vi "BuildCustomDashBoardData.vi"   [LabVIEW 2013]
doc: "This VI builds data and sends it back to the dashboard PC program. By default it sends back the raw values for the first analog, digital, and solenoid module. Modify it to send back the data you want to view. Consider adding higher level data to the Dashboard Datatype.ctl and to this VI. Then update the Dashboard to display the data however you like.\n\nThis software is licensed. Open the labview\\readme\\WPI Robotics Library Open Source License.txt file for more information."
uses:
  <vilib>/Rock Robotics/WPI/DriverStation/WPI_DriverStationDigitalData.ctl
  typedefs/subStates.ctl
  I2C Accelerometer/ADXL345 I2C Axis.ctl
  typedefs/fg_typedef.ctl
  <vilib>/NI_Real-Time Target Support.lvlib
  typedefs/Dashboard Datatype.ctl
  typedefs/DashboardEnable.ctl
  typedefs/custom dash data.ctl
types:
  T1 = typedef "custom dash data.ctl" = cluster{"doubles":cluster{"Front Shooter Speed":dbl, "Arm Rate":dbl, "Arm Distance":dbl, "Right Distance":dbl, "Right Rate":dbl, "Left Rate":dbl, "Left Distance":dbl, "Auger Distance":dbl, "Auger Rate":dbl, "Shooter Bias":dbl, "Rear Shooter Speed":dbl}, "substates":cluster{"Shooter Belt":T2, "Shooter Arm":T2, "Shooter":T2, "Auger ":T2, "Drive":T2}, "bools":cluster{"Auger Safety":bool, "Arm Safety":bool, "Arm Limit":bool}, "Performance":cluster{"CPU Usage":dbl, "Vision mSPI":u32, "Main mSPI":u32}, "Target Info":cluster{"Left":i32, "Top":i32, "Right":i32, "Bottom":i32, "Target CoM X":dbl, "Target CoM Y":dbl}}
  T2 = typedef "subStates.ctl" = enum16{"null", "wait", "driver control", "auto", "manual override", "hold position", "rotate", "pickup", "pass", "load", "goto shoot", "shoot", "end"}
  T3 = typedef "DashboardEnable.ctl" = cluster{"Analog Module 1":bool[], "Analog Module 2":bool[], "Digital Module 1":bool, "Digital Module 2":bool, "Solenoid Module":bool}
  T4 = typedef "Dashboard Datatype.ctl" = cluster{cluster{"AnalogModule[0]":cluster{"Channel[0]":sgl, "Channel[1]":sgl, "Channel[2]":sgl, "Channel[3]":sgl, "Channel[4]":sgl, "Channel[5]":sgl, "Channel[6]":sgl, "Channel[7]":sgl}, "AnalogModule[1]":cluster{"Channel[0]":sgl, "Channel[1]":sgl, "Channel[2]":sgl, "Channel[3]":sgl, "Channel[4]":sgl, "Channel[5]":sgl, "Channel[6]":sgl, "Channel[7]":sgl}}, cluster{"DigitalModule[0]":T5, "DigitalModule[1]":T5}, "Solenoid":u8}
  T5 = typedef "WPI_DriverStationDigitalData.ctl" = cluster{"Relay Fwd":u8, "Relay Rev":u8, "GPIO":u16, "GPIO_OE":u16, "PWM":cluster{"PWM[0]":u8, "PWM[1]":u8, "PWM[2]":u8, "PWM[3]":u8, "PWM[4]":u8, "PWM[5]":u8, "PWM[6]":u8, "PWM[7]":u8, "PWM[8]":u8, "PWM[9]":u8}}
  T6 = cluster{"doubles":cluster{"Shooter Speed":dbl, "Turret Rate":dbl, "Turret Distance":dbl, "Right Distance":dbl, "Right Rate":dbl, "Left Rate":dbl, "Left Distance":dbl, "Ang, Rate":dbl, "Angle":dbl}, "substates":cluster{"Shooter":T2, "Upper Belts":T2, "Lower Belts":T2, "Turret ":T2, "Drive":T2}, "bools":cluster{"VLAD Balakced":bool, "Safety":bool}}
  T7 = typedef "fg_typedef.ctl" = enum16{"Get", "Set"}
  T8 = cluster{"AnalogModule[0]":cluster{"Channel[0]":sgl, "Channel[1]":sgl, "Channel[2]":sgl, "Channel[3]":sgl, "Channel[4]":sgl, "Channel[5]":sgl, "Channel[6]":sgl, "Channel[7]":sgl}, "AnalogModule[1]":cluster{"Channel[0]":sgl, "Channel[1]":sgl, "Channel[2]":sgl, "Channel[3]":sgl, "Channel[4]":sgl, "Channel[5]":sgl, "Channel[6]":sgl, "Channel[7]":sgl}}
  T9 = cluster{"DigitalModule[0]":T5, "DigitalModule[1]":T5}
  T10 = cluster{"Channel[0]":sgl, "Channel[1]":sgl, "Channel[2]":sgl, "Channel[3]":sgl, "Channel[4]":sgl, "Channel[5]":sgl, "Channel[6]":sgl, "Channel[7]":sgl}[]
  T11 = cluster{"Channel[0]":sgl, "Channel[1]":sgl, "Channel[2]":sgl, "Channel[3]":sgl, "Channel[4]":sgl, "Channel[5]":sgl, "Channel[6]":sgl, "Channel[7]":sgl}
  T12 = cluster{"AnalogModule[0][0]":sgl, "AnalogModule[0][1]":sgl, "AnalogModule[0][2]":sgl, "AnalogModule[0][3]":sgl, "AnalogModule[0][4]":sgl, "AnalogModule[0][5]":sgl, "AnalogModule[0][6]":sgl, "AnalogModule[0][7]":sgl}
  T13 = cluster{"[0]":cluster{"Channel[0]":sgl, "Channel[1]":sgl, "Channel[2]":sgl, "Channel[3]":sgl, "Channel[4]":sgl, "Channel[5]":sgl, "Channel[6]":sgl, "Channel[7]":sgl}, "[1]":cluster{"Channel[0]":sgl, "Channel[1]":sgl, "Channel[2]":sgl, "Channel[3]":sgl, "Channel[4]":sgl, "Channel[5]":sgl, "Channel[6]":sgl, "Channel[7]":sgl}}
  T14 = typedef "FPGA_DIODevRef.ctl" = cluster{"DevStatus":errorcluster, "Module":T15}
  T15 = typedef "FPGA_TypedefDigitalModule.ctl" = enum16{"Digital Module 1", "Digital Module 2"}
  T16 = cluster{"[0]":u8, "[1]":u8, "[2]":u8, "[3]":u8, "[4]":u8, "[5]":u8, "[6]":u8, "[7]":u8, "[8]":u8, "[9]":u8}
  T17 = typedef "FPGA_SolenoidDevRef.ctl" = cluster{"DevStatus":errorcluster, "Module":T18}
  T18 = typedef "FPGA_TypedefSolenoidModule.ctl" = enum16{"Solenoid Module 1", "Solenoid Module 2"}
  T19 = cluster{"Front Shooter Speed":dbl, "Arm Rate":dbl, "Arm Distance":dbl, "Right Distance":dbl, "Right Rate":dbl, "Left Rate":dbl, "Left Distance":dbl, "Auger Distance":dbl, "Auger Rate":dbl, "Shooter Bias":dbl, "Rear Shooter Speed":dbl}
  T20 = cluster{"Auger Safety":bool, "Arm Safety":bool, "Arm Limit":bool}
  T21 = cluster{"CPU Usage":dbl, "Vision mSPI":u32, "Main mSPI":u32}
  T22 = cluster{"Left":i32, "Top":i32, "Right":i32, "Bottom":i32, "Target CoM X":dbl, "Target CoM Y":dbl}
  T23 = typedef "WPI_EncoderDevRef.ctl" = cluster{"DevStatus":errorcluster, "EncoderIndex":T24, "CounterIndex":T25, "DistancePerCount":dbl, "Decoding Type":T26}
  T24 = typedef "FPGA_EncoderIdx.ctl" = enum8{"Enc 0", "Enc 1", "Enc 2", "Enc 3", "Invalid"}
  T25 = typedef "FPGA_CounterCtrSystemIndex.ctl" = enum8{"Ctr 0", "Ctr 1", "Ctr 2", "Ctr 3", "Ctr 4", "Ctr 5", "Ctr 6", "Ctr 7", "Invalid"}
  T26 = typedef "WPI_EncoderType.ctl" = enum16{"1x", "2x", "4x"}
  T27 = typedef "ADXL345 I2C Axis.ctl" = u8
  T28 = typedef "WPI_I2CDevRef.ctl" = cluster{"DevStatus":errorcluster, "Digital Module":T15, "Device Address":u8}
  T29 = typedef "WPI_GyroDevRef.ctl" = cluster{"DevStatus":errorcluster, "Analog Module":T30, "Analog Channel":T31, "Offset":dbl, "Gain (VoltsPerDegree/Second)":dbl}
  T30 = typedef "FPGA_TypedefAnalogModule.ctl" = enum16{"Analog Module 1", "Analog Module 2"}
  T31 = typedef "FPGA_AIChannel.ctl" = enum8{"AI 1", "AI 2", "AI 3", "AI 4", "AI 5", "AI 6", "AI 7", "AI 8", "Invalid"}
  T32 = typedef "WPI_MotorControlDeviceRef.ctl" = cluster{"DeviceStatus":errorcluster, "Type":enum16{"PWM", "CAN"}, "PWM":cluster{"Digital Module":T15, "PWM Channel":T33, "DeadBand":T34}, "CAN":cluster{"Device Number":u8, "Control Mode":T35, "Semaphore":T36, "Max Vout":dbl}, "Invert":bool, "TransformRef":T37, "InvTransformRef":T37}
  T33 = typedef "FPGA_DIOPWMChannel.ctl" = enum8{"PWM 1", "PWM 2", "PWM 3", "PWM 4", "PWM 5", "PWM 6", "PWM 7", "PWM 8", "PWM 9", "PWM 10", "Invalid"}
  T34 = typedef "WPI_PWMDeadband.ctl" = cluster{"Name":string, "maxPositivePwm":i32, "minPositivePwm":i32, "centerPwm":i32, "maxNegativePwm":i32, "minNegativePwm":i32, "angularRange":u16}
  T35 = typedef "WPI_CANJaguar_ControlMode.ctl" = enum8{"Percent VBus", "Current", "Speed", "Position", "Voltage"}
  T36 = typedef "Semaphore RefNum" = refnum<k1>
  T37 = typedef "WPI_PWMTransform_ConPane.ctl" = refnum<vi>
  T38 = cluster{"Left":i32, "Top":i32, "Right":i32, "Bottom":i32}
  T39 = typedef "vision data.ctl" = cluster{"x":dbl, "y":dbl, "area":dbl, "width":dbl, "height":dbl, "Hot Goal Present?":bool, "distance":dbl}
  T40 = typedef "NI_Real-Time Target Support.lvlib/RT CPU Load.ctl" = cluster{"Total (%)":dbl, "Time Critical (%)":dbl, "Timed Structures (%)":dbl, "High (%)":dbl, "Above Normal (%)":dbl, "Normal (%)":dbl, "Background (%)":dbl, "Idle (%)":dbl, "ISR (%)":dbl}
  T41 = cluster{"Vision mSPI":u32, "Main mSPI":u32, "Dash mSPI":u32}
  T42 = cluster{"VLAD Balance":bool, "Safety":bool, "Turret Limit":bool}
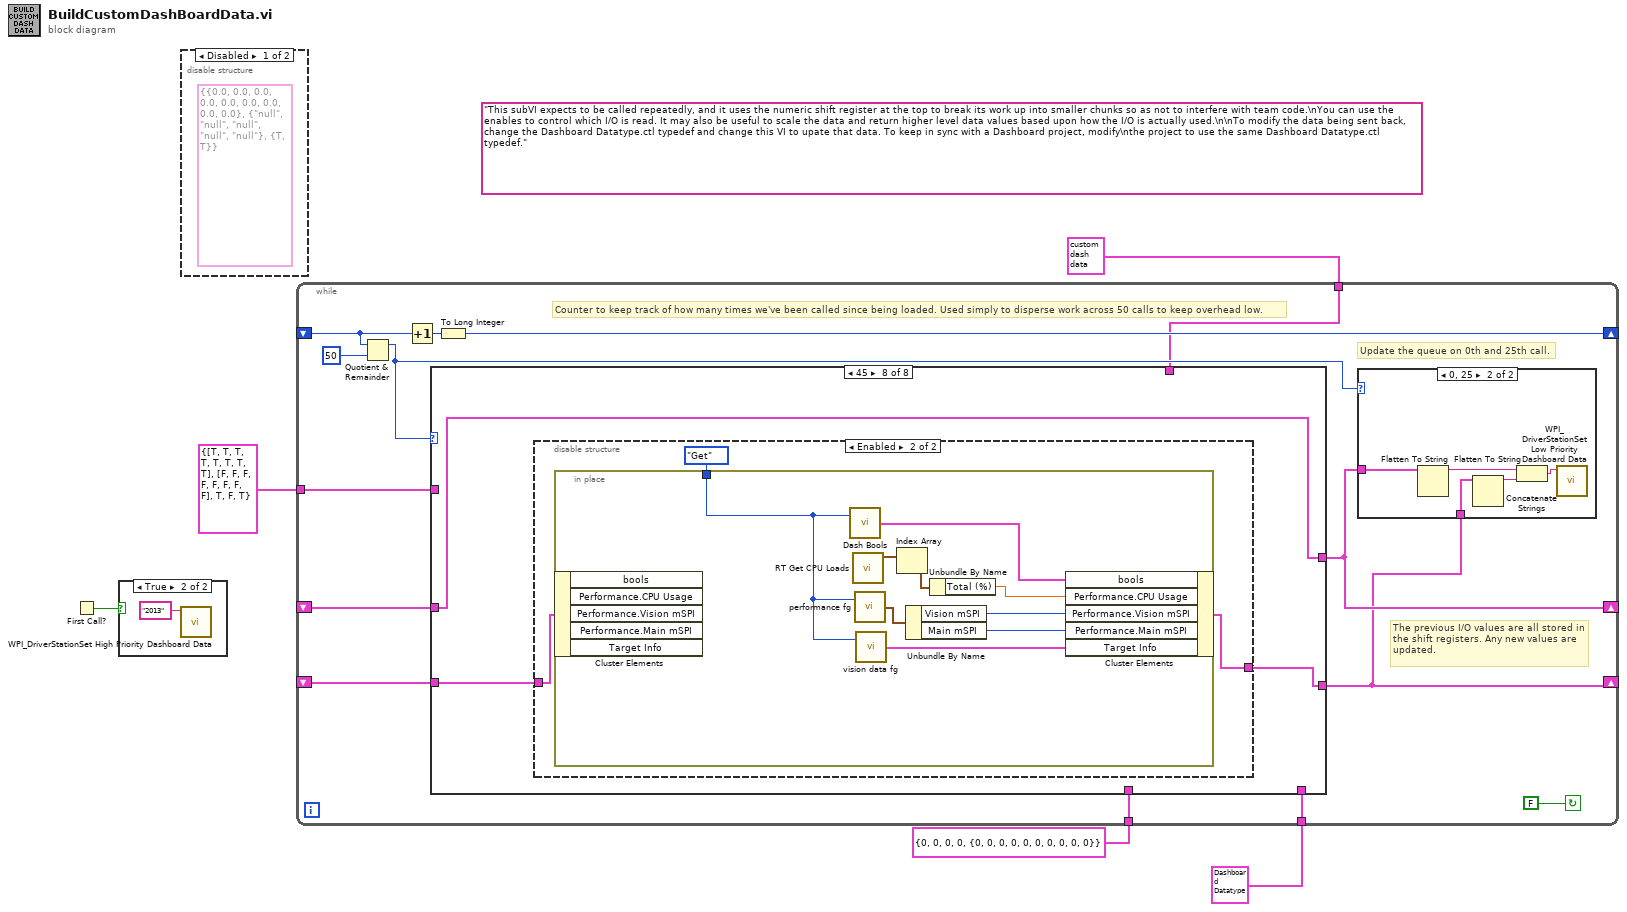
[diagram p0: block diagram]
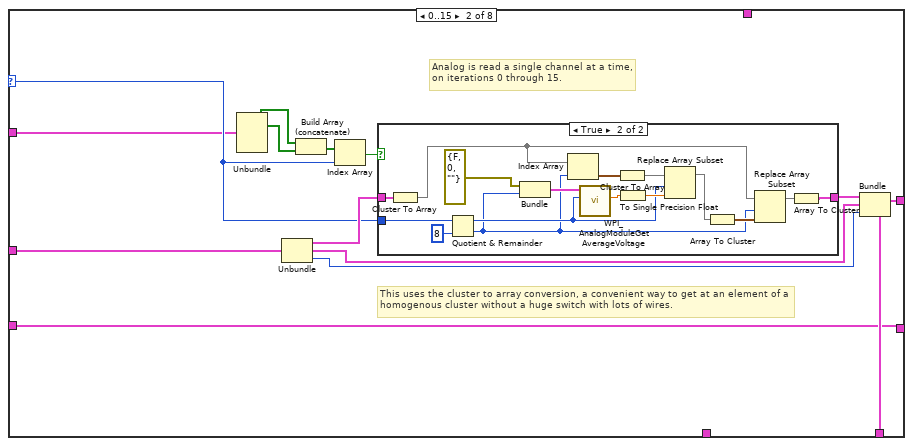
[diagram p6: hidden frame]
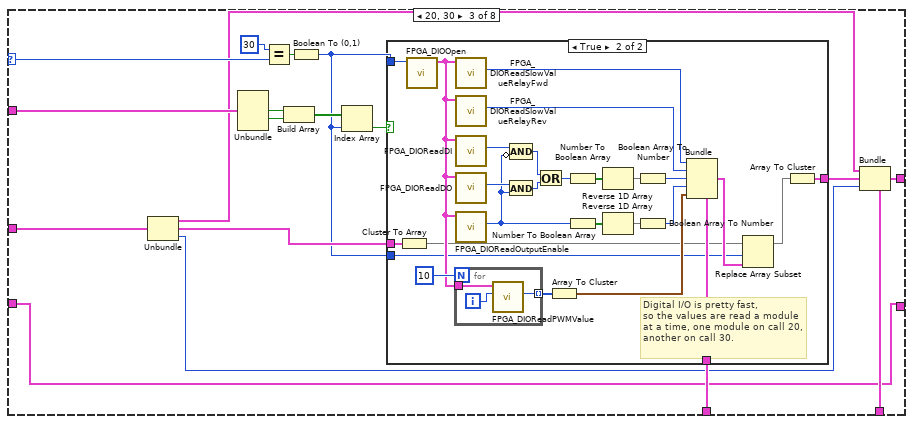
[diagram p8: hidden frame]
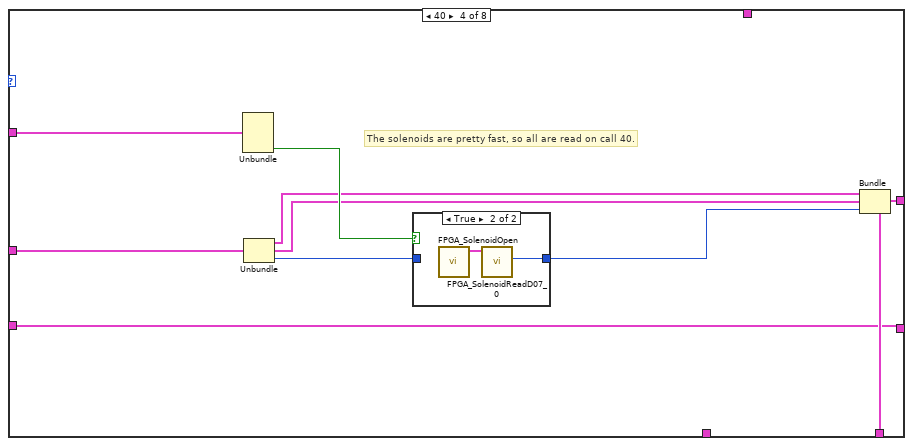
[diagram p10: hidden frame]
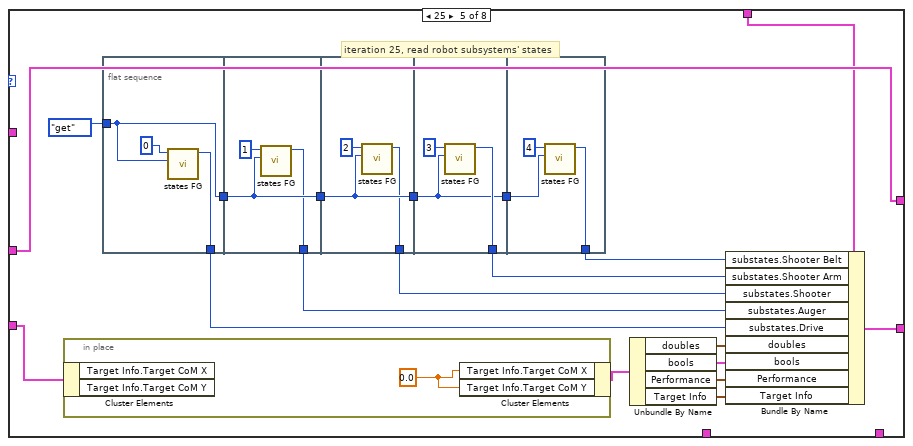
[diagram p12: hidden frame]
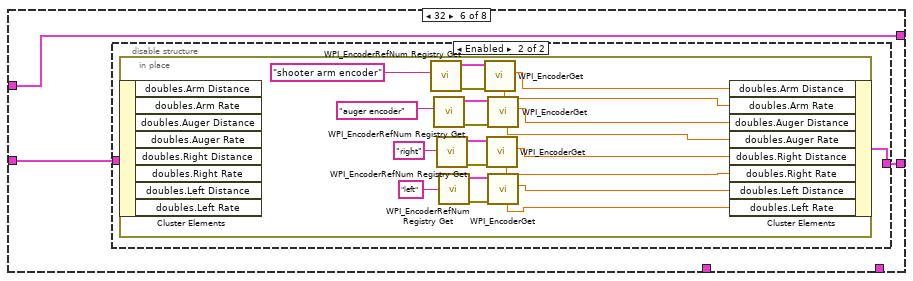
[diagram p13: hidden frame]
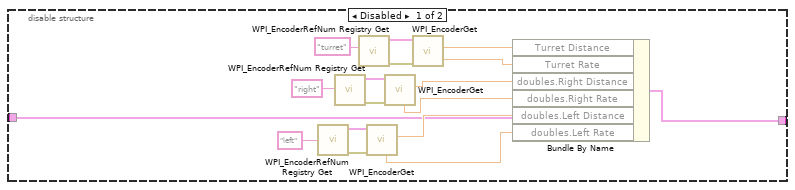
[diagram p14: hidden frame]
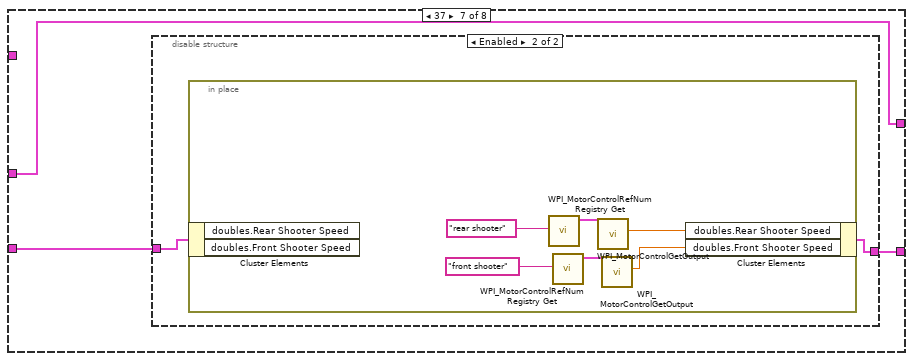
[diagram p15: hidden frame]
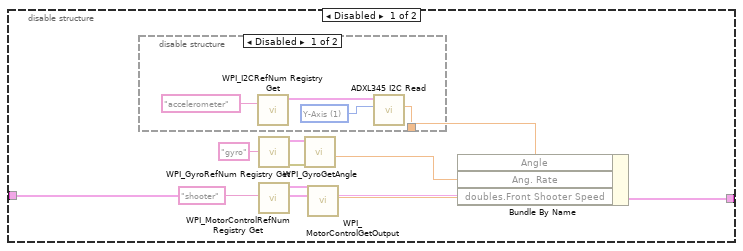
[diagram p16: hidden frame]
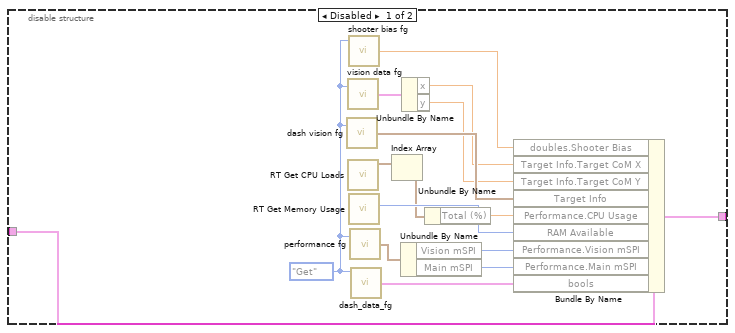
[diagram p18: hidden frame]
diagram:
  (unwired) "This subVI expects to be called repeatedly, and it uses the numeric shift register at the top to break its work up into smaller chunks so as not to interfere with team code.\nYou can use the enables to control which I/O is read. It may also be useful to scale the data and return higher level data values based upon how the I/O is actually used.\n\nTo modify the data being sent back, change the Dashboard Datatype.ctl typedef and change this VI to upate that data. To keep in sync with a Dashboard project, modify\nthe project to use the same Dashboard Datatype.ctl typedef."
  n1 = First Call?() -> (First Call?: T/F=w3:bool)
  n2 = case shown="True" w3 {
    frame False {
    }
    frame True {
      n3 = call <vilib>:"WPI_DriverStationSet High Priority Dashboard Data.vi"("User Data"="2013") -> ()  [unwired: 10 in, 1 out]
    }
  }
  n4 = disable-structure shown="Disabled" {
    frame Disabled {
      (unwired) T6 {"doubles"={"Shooter Speed"=0.0, "Turret Rate"=0.0, "Turret Distance"=0.0, "Right Distance"=0.0, "Right Rate"=0.0, "Left Rate"=0.0, "Left Distance"=0.0, "Ang, Rate"=0.0, "Angle"=0.0}, "substates"={"Shooter"=enum."null", "Upper Belts"=enum."null", "Lower Belts"=enum."null", "Turret "=enum."null", "Drive"=enum."null"}, "bools"={"VLAD Balakced"=TRUE, "Safety"=TRUE}}
    }
    frame Enabled {
    }
  }
  n5 = while {
    shift-right: [w13] -> _
    shift-left: _ -> [w15]
    shift-right: [w10] -> _
    shift-left: _ -> [w18]
    tunnel: T5 {"Relay Fwd"=0, "Relay Rev"=0, "GPIO"=0, "GPIO_OE"=0, "PWM"={"PWM[0]"=0, "PWM[1]"=0, "PWM[2]"=0, "PWM[3]"=0, "PWM[4]"=0, "PWM[5]"=0, "PWM[6]"=0, "PWM[7]"=0, "PWM[8]"=0, "PWM[9]"=0}} ("DigitalModule[1]") -> [w17]
    tunnel: T4 {{"AnalogModule[0]"={"Channel[0]"=0.0, "Channel[1]"=0.0, "Channel[2]"=0.0, "Channel[3]"=0.0, "Channel[4]"=0.0, "Channel[5]"=0.0, "Channel[6]"=0.0, "Channel[7]"=0.0}, "AnalogModule[1]"={"Channel[0]"=0.0, "Channel[1]"=0.0, "Channel[2]"=0.0, "Channel[3]"=0.0, "Channel[4]"=0.0, "Channel[5]"=0.0, "Channel[6]"=0.0, "Channel[7]"=0.0}}, {"DigitalModule[0]"={"Relay Fwd"=0, "Relay Rev"=0, "GPIO"=0, "GPIO_OE"=0, "PWM"={"PWM[0]"=0, "PWM[1]"=0, "PWM[2]"=0, "PWM[3]"=0, "PWM[4]"=0, "PWM[5]"=0, "PWM[6]"=0, "PWM[7]"=0, "PWM[8]"=0, "PWM[9]"=0}}, "DigitalModule[1]"={"Relay Fwd"=0, "Relay Rev"=0, "GPIO"=0, "GPIO_OE"=0, "PWM"={"PWM[0]"=0, "PWM[1]"=0, "PWM[2]"=0, "PWM[3]"=0, "PWM[4]"=0, "PWM[5]"=0, "PWM[6]"=0, "PWM[7]"=0, "PWM[8]"=0, "PWM[9]"=0}}}, "Solenoid"=0} ("Dashboard Data") -> [w12]
    tunnel: T3 {"Analog Module 1"=[TRUE, TRUE, TRUE, TRUE, TRUE, TRUE, TRUE, TRUE], "Analog Module 2"=[FALSE, FALSE, FALSE, FALSE, FALSE, FALSE, FALSE, FALSE], "Digital Module 1"=TRUE, "Digital Module 2"=FALSE, "Solenoid Module"=TRUE} ("Dashboard Enables") -> [w11]
    shift-right: [w7] -> _
    shift-left: _ -> [w8]
    tunnel: T1 {"doubles"={"Front Shooter Speed"=0.0, "Arm Rate"=0.0, "Arm Distance"=0.0, "Right Distance"=0.0, "Right Rate"=0.0, "Left Rate"=0.0, "Left Distance"=0.0, "Auger Distance"=0.0, "Auger Rate"=0.0, "Shooter Bias"=0.0, "Rear Shooter Speed"=0.0}, "substates"={"Shooter Belt"=enum."null", "Shooter Arm"=enum."null", "Shooter"=enum."null", "Auger "=enum."null", "Drive"=enum."null"}, "bools"={"Auger Safety"=FALSE, "Arm Safety"=FALSE, "Arm Limit"=FALSE}, "Performance"={"CPU Usage"=0.0, "Vision mSPI"=0, "Main mSPI"=0}, "Target Info"={"Left"=0, "Top"=0, "Right"=0, "Bottom"=0, "Target CoM X"=0.0, "Target CoM Y"=0.0}} ("Custom Dash Data") -> [w9]
    stop <- FALSE continue-if-true
    # "Counter to keep track of how many times we've been called since being loaded. Used simply to disperse work across 50 calls to keep overhead low."
    # "Update the queue on 0th and 25th call."
    # "The previous I/O values are all stored in\nthe shift registers. Any new values are\nupdated."
    n6 = Quotient & Remainder(x=w15, y=50) -> (x-y*floor(x/y)=w14:i32)  [unwired: 1 out]
    n7 = Increment(x=w15) -> (x+1=w20:i32)
    n8 = case shown="45" w14 {
      selector: w14 -> [_ w36 w72 _ _ _ _ _]
      tunnel: [w27 w32 w63 w113 w128 w156 w199 w223] -> w10
      tunnel: w18 -> [w27 w31 w65 w115 w128 w156 w199 w223]
      tunnel: w17 -> [_ _ w76 _ _ _ _ _]
      tunnel: w12 -> [_ w38 w64 w112 _ _ _ _]
      tunnel: w11 -> [_ w35 w70 w116 _ _ _ _]
      tunnel: w9 -> [_ _ _ _ w126 _ _ _]
      tunnel: [w26 w30 w61 w109 w127 w157 w198 w224] -> w7
      tunnel: w8 -> [w26 w30 w61 w109 w121 w155 w197 w222]
      frame Default {
        # "Don't update any I/O"
      }
      frame 0..15 {
        # "This uses the cluster to array conversion, a convenient way to get at an element of a\nhomogenous cluster without a huge switch with lots of wires."
        # "Analog is read a single channel at a time,\non iterations 0 through 15."
        n9 = Unbundle(w35) -> ("Analog Module 1"=w34:bool[], "Analog Module 2"=w33:bool[])  [unwired: 3 out]
        n10 = Unbundle(w31) -> (w37:T8, w29:T9, "Solenoid"=w28:u8)
        n11 = Build Array (concatenate)(w34, w33) -> (w40:bool[])
        n12 = Index Array(array=w40, index=w36) -> (element=w41:bool)
        n13 = case shown="True" w41 {
          tunnel: w36 -> [_ w49]
          tunnel: [w42 w46] -> w39
          tunnel: w37 -> [w42 w45]
          frame False {
          }
          frame True {
            n14 = Cluster To Array(cluster=w45) -> (array=w44:T10)
            n15 = Quotient & Remainder(x=w49, y=8) -> (x-y*floor(x/y)=w48:i32, floor(x/y)=w43:i32)
            n16 = Bundle("DevStatus"=errorcluster {"status"=FALSE, "code"=0, "source"=""}, w43) -> (w57:cluster{"DevStatus":errorcluster, i32})  [unwired: 1 out]
            n17 = Index Array(array=w44, index=w43) -> (element=w51:T11)
            n18 = call <vilib>:"WPI_AnalogModuleGetAverageVoltage.vi"("Channel"=w48, "AnalogModuleDevStatus"=w57) -> ("Average Voltage"=w54:dbl)  [unwired: 1 in, 8 out]
            n19 = Cluster To Array(cluster=w51) -> (array=w50:sgl[])
            n20 = To Single Precision Float(number=w54) -> (single precision float=w53:sgl)
            n21 = Replace Array Subset(array=w50, new element=w53, index=w48) -> (w52:sgl[])
            n22 = Array To Cluster(array=w52) -> (cluster=w56:T12)
            n23 = Replace Array Subset(array=w44, new element=w56, index=w43) -> (w47:T10)
            n24 = Array To Cluster(array=w47) -> (cluster=w46:T13)
          }
        }
        n25 = Bundle(cluster=w38, w39, w29, "Solenoid"=w28) -> (w32:T4)
      }
      frame 20, 30 {
        n26 = Unbundle(w65) -> (w60:T8, w67:T9, "Solenoid"=w59:u8)
        n27 = Unbundle(w70) -> ("Digital Module 1"=w69:bool, "Digital Module 2"=w68:bool)  [unwired: 3 out]
        n28 = Equal?(x=30, y=w72) -> (x = y?=w74:bool)
        n29 = Build Array(w69, w68) -> (w71:bool[])
        n30 = Boolean To (0,1)(Boolean=w74) -> (0, 1=w62:i16)
        n31 = Index Array(array=w71, index=w62) -> (element=w73:bool)
        n32 = case shown="True" w73 {
          tunnel: w76 -> [_ w85]
          tunnel: [w77 w78] -> w66
          tunnel: w62 -> [_ w83]
          tunnel: w62 -> [_ w82]
          tunnel: w67 -> [w77 w81]
          frame False {
          }
          frame True {
            # "Digital I/O is pretty fast,\nso the values are read a module\nat a time, one module on call 20,\nanother on call 30."
            n33 = Cluster To Array(cluster=w81) -> (array=w80:T5[])
            n34 = call <vilib>:"FPGA_DIOOpen.vi"("Module (Module 1)"=w83) -> ("DIODeviceRef"=w101:T14)  [unwired: 1 in, 9 out]
            n35 = for {
              N: 10 -> [_]
              tunnel: w101 -> [w106]
              tunnel: [w104] -> w102 mode=indexing
              i -> [w105]
              n36 = call <vilib>:"FPGA_DIOReadPWMValue.vi"("PWMChannel"=w105, "DIODeviceRef In"=w106) -> ("PWMValue"=w104:u8)  [unwired: 1 in, 8 out]
            }
            n37 = call <vilib>:"FPGA_DIOReadSlowValueRelayFwd.vi"("DIODeviceRef In"=w101) -> ("Relay Forward"=w94:u8)  [unwired: 1 in, 9 out]
            n38 = call <vilib>:"FPGA_DIOReadSlowValueRelayRev.vi"("DIODeviceRef In"=w101) -> ("Relay Reverse"=w95:u8)  [unwired: 1 in, 9 out]
            n39 = call <vilib>:"FPGA_DIOReadDI.vi"("DIODeviceRef In"=w101) -> ("DI"=w99:u16)  [unwired: 1 in, 9 out]
            n40 = call <vilib>:"FPGA_DIOReadDO.vi"("DIODeviceRef In"=w101) -> ("DO"=w98:u16)  [unwired: 1 in, 9 out]
            n41 = call <vilib>:"FPGA_DIOReadOutputEnable.vi"("DIODeviceRef In"=w101) -> ("OutputEnable"=w89:u16)  [unwired: 1 in, 9 out]
            n42 = And(x=w98, y=w89) -> (x .and. y?=w97:u16)
            n43 = Compound Arithmetic op=AND(w99, invert w89) -> (w96:u16)
            n44 = Or(x=w96, y=w97) -> (x .or. y?=w87:u16)
            n45 = Array To Cluster(array=w102) -> (cluster=w100:T16)
            n46 = Number To Boolean Array(number=w87) -> (Boolean array=w92:bool[])
            n47 = Number To Boolean Array(number=w89) -> (Boolean array=w91:bool[])
            n48 = Reverse 1D Array(array=w92) -> (reversed array=w93:bool[])
            n49 = Reverse 1D Array(array=w91) -> (reversed array=w90:bool[])
            n50 = Boolean Array To Number(Boolean array=w93) -> (number=w86:u32)
            n51 = Boolean Array To Number(Boolean array=w90) -> (number=w88:u32)
            n52 = Bundle(cluster=w85, "Relay Fwd"=w94, "Relay Rev"=w95, "GPIO"=w86, "GPIO_OE"=w88, "PWM"=w100) -> (w84:T5)
            n53 = Replace Array Subset(array=w80, new element=w84, index=w82) -> (w79:T5[])
            n54 = Array To Cluster(array=w79) -> (cluster=w78:cluster{"[0]":T5, "[1]":T5})
          }
        }
        n55 = Bundle(cluster=w64, w60, w66, "Solenoid"=w59) -> (w63:T4)
      }
      frame 40 {
        # "The solenoids are pretty fast, so all are read on call 40."
        n56 = Unbundle(w116) -> ("Solenoid Module"=w110:bool)  [unwired: 4 out]
        n57 = Unbundle(w115) -> (w108:T8, w107:T9, "Solenoid"=w114:u8)
        n58 = case shown="True" w110 {
          tunnel: [w117 w118] -> w111
          tunnel: w114 -> [w117 _]
          frame False {
          }
          frame True {
            n59 = call <vilib>:"FPGA_SolenoidOpen.vi"() -> ("SolenoidDevRef"=w119:T17)  [unwired: 2 in, 9 out]
            n60 = call <vilib>:"FPGA_SolenoidReadD07_0.vi"("SolenoidDevRef"=w119) -> ("DO7:0"=w118:u8)  [unwired: 1 in, 9 out]
          }
        }
        n61 = Bundle(cluster=w112, w108, w107, "Solenoid"=w111) -> (w113:T4)
      }
      frame 25 {
        # "iteration 25, read robot subsystems' states"
        n62 = in-place {
          w139 = 0.0
          n63 = in-place-cluster #1(w121) -> ()  [unwired: 2 out]
          n64 = in-place-cluster #1("Target Info.Target CoM X"=w139, "Target Info.Target CoM Y"=w139) -> (w120:T1)
        }
        n65 = flat-sequence {
          tunnel: enum16{"set", "get"}."get" ("menu (get)") -> [w142]
          tunnel: [w142] -> w135
          tunnel: [w140] -> w129
          tunnel: [w145] -> w136
          tunnel: w135 -> [w145]
          tunnel: [w143] -> w130
          tunnel: [w148] -> w137
          tunnel: w136 -> [w148]
          tunnel: [w146] -> w131
          tunnel: w137 -> [w149]
          tunnel: [w150] -> w132
          tunnel: [w149] -> w134
          tunnel: w134 -> [w153]
          tunnel: [w152] -> w133
          frame #0 {
            n66 = call "states FG.vi"("menu (get)"=w142, "Loop ID"=0) -> ("subState out"=w140:T2)  [unwired: 6 in, 3 out]
          }
          frame #1 {
            n67 = call "states FG.vi"("menu (get)"=w145, "Loop ID"=1) -> ("subState out"=w143:T2)  [unwired: 6 in, 3 out]
          }
          frame #2 {
            n68 = call "states FG.vi"("menu (get)"=w148, "Loop ID"=2) -> ("subState out"=w146:T2)  [unwired: 6 in, 3 out]
          }
          frame #3 {
            n69 = call "states FG.vi"("menu (get)"=w149, "Loop ID"=3) -> ("subState out"=w150:T2)  [unwired: 6 in, 3 out]
          }
          frame #4 {
            n70 = call "states FG.vi"("menu (get)"=w153, "Loop ID"=4) -> ("subState out"=w152:T2)  [unwired: 6 in, 3 out]
          }
        }
        n71 = Unbundle By Name(w120) -> ("doubles"=w125:T19, "bools"=w124:T20, "Performance"=w123:T21, "Target Info"=w122:T22)
        n72 = Bundle By Name(cluster=w126, "substates.Shooter Belt"=w133, "substates.Shooter Arm"=w132, "substates.Shooter"=w131, "substates.Auger"=w130, "substates.Drive"=w129, "doubles"=w125, "bools"=w124, "Performance"=w123, "Target Info"=w122) -> (w127:T1)
      }
      frame 32 {
        n73 = disable-structure shown="Enabled" {
          disable-tunnel: [w174 w175] -> w157
          disable-tunnel: w155 -> [w158 w176]
          frame Disabled {
            n74 = call <vilib>:"WPI_EncoderRefNum Registry Get.vi"("refnum name"="left") -> ("error out"=w170:errorcluster, "EncoderDevRef"=w169:T23)  [unwired: 9 in]
            n75 = call <vilib>:"WPI_EncoderRefNum Registry Get.vi"("refnum name"="right") -> ("error out"=w168:errorcluster, "EncoderDevRef"=w167:T23)  [unwired: 9 in]
            n76 = call <vilib>:"WPI_EncoderRefNum Registry Get.vi"("refnum name"="turret") -> ("error out"=w166:errorcluster, "EncoderDevRef"=w165:T23)  [unwired: 9 in]
            n77 = call <vilib>:"WPI_EncoderGet.vi"("error in (no error)"=w170, "EncoderDevRef"=w169) -> ("Distance"=w160:dbl, "Rate"=w159:dbl)  [unwired: 4 in, 4 out]
            n78 = call <vilib>:"WPI_EncoderGet.vi"("error in (no error)"=w168, "EncoderDevRef"=w167) -> ("Distance"=w162:dbl, "Rate"=w161:dbl)  [unwired: 4 in, 4 out]
            n79 = call <vilib>:"WPI_EncoderGet.vi"("error in (no error)"=w166, "EncoderDevRef"=w165) -> ("Distance"=w164:dbl, "Rate"=w163:dbl)  [unwired: 4 in, 4 out]
            n80 = Bundle By Name(cluster=w158, "Turret Distance"=w164, "Turret Rate"=w163, "doubles.Right Distance"=w162, "doubles.Right Rate"=w161, "doubles.Left Distance"=w160, "doubles.Left Rate"=w159) -> (w174:T1)
          }
          frame Enabled {
            n81 = in-place {
              n82 = in-place-cluster #2(w176) -> ()  [unwired: 8 out]
              n83 = call <vilib>:"WPI_EncoderRefNum Registry Get.vi"("refnum name"="shooter arm encoder") -> ("error out"=w180:errorcluster, "EncoderDevRef"=w181:T23)  [unwired: 9 in]
              n84 = call <vilib>:"WPI_EncoderRefNum Registry Get.vi"("refnum name"="auger encoder") -> ("error out"=w190:errorcluster, "EncoderDevRef"=w189:T23)  [unwired: 9 in]
              n85 = call <vilib>:"WPI_EncoderRefNum Registry Get.vi"("refnum name"="right") -> ("error out"=w192:errorcluster, "EncoderDevRef"=w191:T23)  [unwired: 9 in]
              n86 = call <vilib>:"WPI_EncoderRefNum Registry Get.vi"("refnum name"="left") -> ("error out"=w194:errorcluster, "EncoderDevRef"=w193:T23)  [unwired: 9 in]
              n87 = call <vilib>:"WPI_EncoderGet.vi"("error in (no error)"=w180, "EncoderDevRef"=w181) -> ("Distance"=w179:dbl, "Rate"=w178:dbl)  [unwired: 4 in, 4 out]
              n88 = call <vilib>:"WPI_EncoderGet.vi"("error in (no error)"=w192, "EncoderDevRef"=w191) -> ("Distance"=w186:dbl, "Rate"=w185:dbl)  [unwired: 4 in, 4 out]
              n89 = call <vilib>:"WPI_EncoderGet.vi"("error in (no error)"=w190, "EncoderDevRef"=w189) -> ("Distance"=w188:dbl, "Rate"=w187:dbl)  [unwired: 4 in, 4 out]
              n90 = call <vilib>:"WPI_EncoderGet.vi"("error in (no error)"=w194, "EncoderDevRef"=w193) -> ("Distance"=w184:dbl, "Rate"=w183:dbl)  [unwired: 4 in, 4 out]
              n91 = in-place-cluster #2("doubles.Arm Distance"=w179, "doubles.Arm Rate"=w178, "doubles.Auger Distance"=w188, "doubles.Auger Rate"=w187, "doubles.Right Distance"=w186, "doubles.Right Rate"=w185, "doubles.Left Distance"=w184, "doubles.Left Rate"=w183) -> (w175:T1)
            }
          }
        }
      }
      frame 37 {
        n92 = disable-structure shown="Enabled" {
          disable-tunnel: [w209 w214] -> w198
          disable-tunnel: w197 -> [w200 w215]
          frame Disabled {
            n93 = disable-structure shown="Disabled" {
              disable-tunnel: [w210 _] -> w204
              frame Disabled {
                w211 = T27 1 items=["X-Axis", "Y-Axis", "Z-Axis"] ("Axis")
                n94 = call <vilib>:"WPI_I2CRefNum Registry Get.vi"("refnum name"="accelerometer") -> ("I2CDevRef"=w212:T28)  [unwired: 9 in, 1 out]
                n95 = call "ADXL345 I2C Read.vi"("Axis"=w211, "I2CDevRef"=w212) -> ("Acceleration"=w210:dbl)  [unwired: 7 in, 2 out]
              }
              frame Enabled {
              }
            }
            n96 = call <vilib>:"WPI_GyroRefNum Registry Get.vi"("refnum name"="gyro") -> ("error out"=w203:errorcluster, "GyroDevRef"=w202:T29)  [unwired: 9 in]
            n97 = call <vilib>:"WPI_MotorControlRefNum Registry Get.vi"("refnum name"="shooter") -> ("MotorControlDevRef"=w207:T32)  [unwired: 9 in, 1 out]
            n98 = call <vilib>:"WPI_GyroGetAngle.vi"("error in (no error)"=w203, "GyroDevRef"=w202) -> ("Angular Rate"=w201:dbl)  [unwired: 6 in, 3 out]
            n99 = call <vilib>:"WPI_MotorControlGetOutput.vi"("MotorControlDevRef"=w207) -> ("Output"=w206:dbl)  [unwired: 8 in, 2 out]
            n100 = Bundle By Name(cluster=w200, "Angle"=w204, "Ang. Rate"=w201, "doubles.Front Shooter Speed"=w206) -> (w209:T1)
          }
          frame Enabled {
            n101 = in-place {
              n102 = in-place-cluster #3(w215) -> ()  [unwired: 2 out]
              n103 = call <vilib>:"WPI_MotorControlRefNum Registry Get.vi"("refnum name"="rear shooter") -> ("MotorControlDevRef"=w217:T32)  [unwired: 9 in, 1 out]
              n104 = call <vilib>:"WPI_MotorControlRefNum Registry Get.vi"("refnum name"="front shooter") -> ("MotorControlDevRef"=w221:T32)  [unwired: 9 in, 1 out]
              n105 = call <vilib>:"WPI_MotorControlGetOutput.vi"("MotorControlDevRef"=w217) -> ("Output"=w216:dbl)  [unwired: 8 in, 2 out]
              n106 = call <vilib>:"WPI_MotorControlGetOutput.vi"("MotorControlDevRef"=w221) -> ("Output"=w219:dbl)  [unwired: 8 in, 2 out]
              n107 = in-place-cluster #3("doubles.Rear Shooter Speed"=w216, "doubles.Front Shooter Speed"=w219) -> (w214:T1)
            }
          }
        }
      }
      frame 45 {
        n108 = disable-structure shown="Enabled" {
          disable-tunnel: [w240 w241] -> w224
          disable-tunnel: w222 -> [w225 w243]
          frame Disabled {
            w227 = fg_typedef."Get" ("Menu (Get)")
            n109 = call "dash vision fg.vi"("Menu"=w227) -> ("Output"=w231:T38)  [unwired: 1 in]
            n110 = call "vision data fg.vi"("Menu"=w227) -> ("Output"=w230:T39)  [unwired: 1 in]
            n111 = call <vilib>:"RT Get CPU Loads.vi"() -> ("CPU loads"=w234:T40[])  [unwired: 10 in, 1 out]
            n112 = call "shooter bias fg.vi"("Menu"=w227) -> ("output"=w226:dbl)  [unwired: 2 in]
            n113 = call <vilib>:"RT Get Memory Usage.vi"() -> ("available (bytes)"=w235:u32)  [unwired: 8 in, 3 out]
            n114 = call "performance fg.vi"("Menu"=w227) -> ("Output"=w238:T41)  [unwired: 1 in]
            n115 = call "dash_data_fg.vi"("Menu (Get)"=w227) -> ("Output"=w239:T42)  [unwired: 2 in]
            n116 = Index Array(array=w234) -> (element=w233:T40)  [unwired: 1 in]
            n117 = Unbundle By Name(w238) -> ("Vision mSPI"=w236:u32, "Main mSPI"=w237:u32)
            n118 = Unbundle By Name(w230) -> ("x"=w229:dbl, "y"=w228:dbl)
            n119 = Unbundle By Name(w233) -> ("Total (%)"=w232:dbl)
            n120 = Bundle By Name(cluster=w225, "doubles.Shooter Bias"=w226, "Target Info.Target CoM X"=w229, "Target Info.Target CoM Y"=w228, "Target Info"=w231, "Performance.CPU Usage"=w232, "RAM Available"=w235, "Performance.Vision mSPI"=w236, "Performance.Main mSPI"=w237, "bools"=w239) -> (w240:T1)
          }
          frame Enabled {
            n121 = in-place {
              in-place-border: fg_typedef."Get" ("Menu (Get)") -> [w246]
              n122 = in-place-cluster #4(w243) -> ()  [unwired: 5 out]
              n123 = call "Dash Bools.vi"("Menu"=w246) -> ("Output"=w245:T20)  [unwired: 1 in]
              n124 = call <vilib>:"RT Get CPU Loads.vi"() -> ("CPU loads"=w251:T40[])  [unwired: 10 in, 1 out]
              n125 = call "performance fg.vi"("Menu"=w246) -> ("Output"=w247:T41)  [unwired: 1 in]
              n126 = call "vision data fg.vi"("Menu"=w246) -> ("Output"=w244:T39)  [unwired: 1 in]
              n127 = Index Array(array=w251) -> (element=w252:T40)  [unwired: 1 in]
              n128 = Unbundle By Name(w247) -> ("Vision mSPI"=w249:u32, "Main mSPI"=w248:u32)
              n129 = Unbundle By Name(w252) -> ("Total (%)"=w250:dbl)
              n130 = in-place-cluster #4("bools"=w245, "Performance.CPU Usage"=w250, "Performance.Vision mSPI"=w249, "Performance.Main mSPI"=w248, "Target Info"=w244) -> (w241:T1)
            }
          }
        }
      }
    }
    n131 = To Long Integer(number=w20) -> (32bit integer=w13:i32)
    n132 = case shown="0, 25" w14 {
      tunnel: w10 -> [_ w25]
      tunnel: w7 -> [_ w23]
      frame Default {
      }
      frame 0, 25 {
        n133 = Flatten To String(anything=w25) -> (data string=w24:string)  [unwired: 1 in, 4 out]
        n134 = Flatten To String(anything=w23) -> (data string=w21:string)  [unwired: 1 in, 4 out]
        n135 = Concatenate Strings(w24, w21) -> (w22:string)
        n136 = call <vilib>:"WPI_DriverStationSet Low Priority Dashboard Data.vi"("User Data"=w22) -> ()  [unwired: 1 in, 10 out]
      }
    }
  }
